vi "1.vi"() -> ()   [LabVIEW 2015]
panel:
  out "数据":string
  in  "文件路径":path
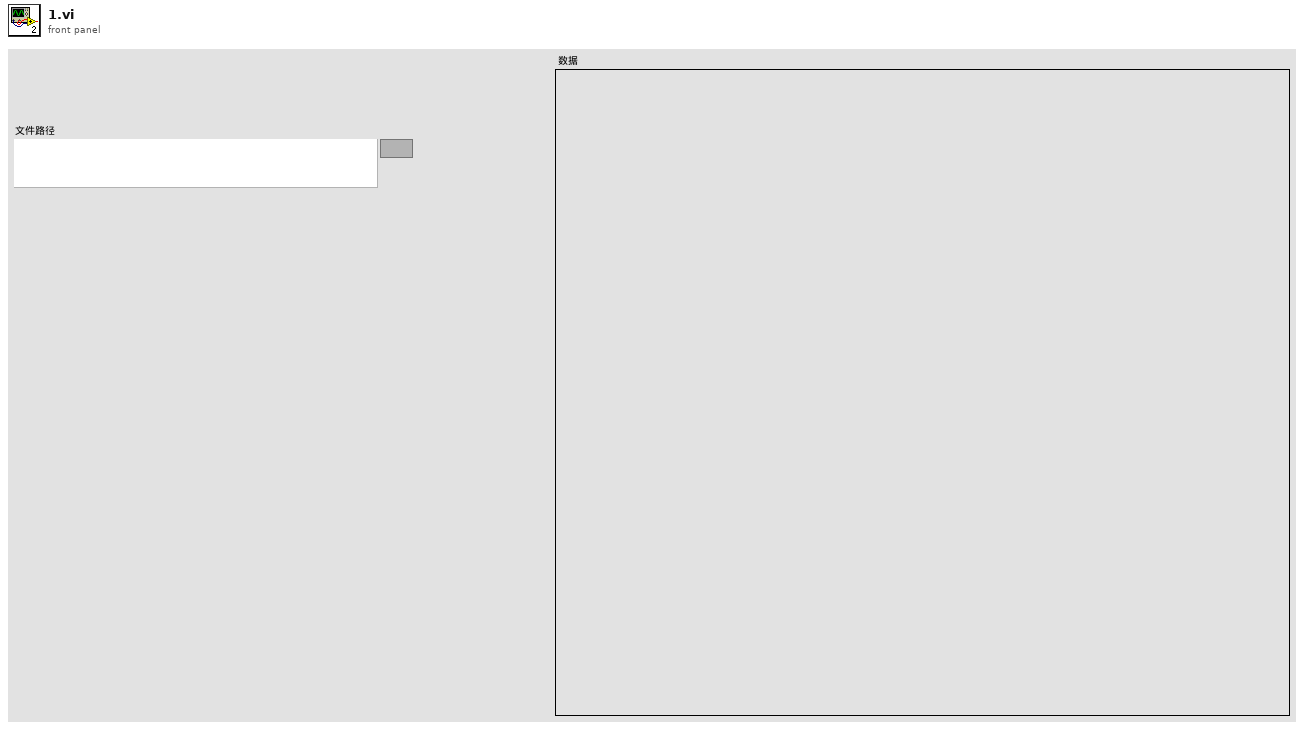
[diagram p1: front panel]
types:
  T1 = enum16{"open", "replace", "create", "open or create", "replace or create", "replace or create with confirmation"}
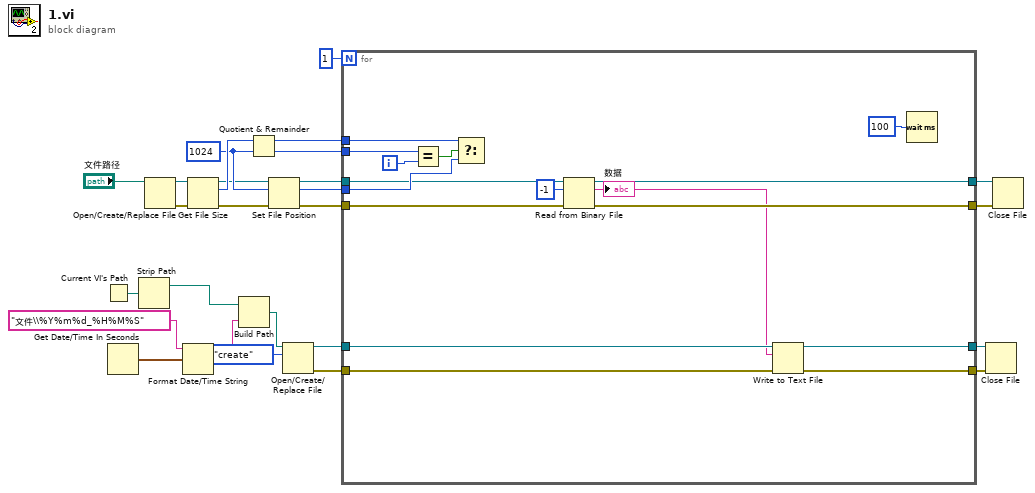
[diagram p0: block diagram]
diagram:
  w19 = 1024 ("y")
  n1 = Current VI's Path() -> (path=w9:path)
  n2 = Get Date/Time In Seconds() -> (seconds since 1Jan1904=w10:timestamp)
  n3 = Strip Path(path=w9) -> (stripped path=w8:path)  [unwired: 1 out]
  n4 = Open/Create/Replace File(file path (use dialog)="文件路径") -> (refnum out=w21:refnum<file>, error out=w22:errorcluster)  [unwired: 5 in, 1 out]
  n5 = Format Date/Time String(time format string (%c)="文件\\%Y%m%d_%H%M%S" ("时间格式字符串(%c)"), seconds (now)=w10) -> (date/time string=w7:string)  [unwired: 1 in]
  n6 = Get File Size(file=w21, error in=w22) -> (refnum out=w14:refnum<file>, size (in bytes)=w20:i64, 0:w13:errorcluster)
  n7 = Build Path(base path=w8, name or relative path=w7) -> (appended path=w6:path)
  n8 = Quotient & Remainder(x=w20, y=w19) -> (x-y*floor(x/y)=w17:i64, floor(x/y)=w18:i64)
  n9 = Set File Position(refnum=w14, error in=w13) -> (refnum out=w12:refnum<file>, error out=w11:errorcluster)  [unwired: 2 in]
  n10 = Open/Create/Replace File(file path (use dialog)=w6, operation (0:open)=T1."create" ("操作(0:open)")) -> (refnum out=w3:refnum<file>, error out=w2:errorcluster)  [unwired: 4 in, 1 out]
  n11 = for {
    N: 1 -> [_]
    tunnel: w12 -> [w28]
    tunnel: w11 -> [w27]
    tunnel: [w41] -> w25
    tunnel: [w40] -> w24
    tunnel: w19 -> [w35]
    tunnel: w18 -> [w39]
    tunnel: w17 -> [w36]
    tunnel: [w32] -> w15
    tunnel: [w33] -> w16
    tunnel: w3 -> [w31]
    tunnel: w2 -> [w30]
    i -> [w38]
    n12 = Equal?(x=w39, y=w38) -> (x = y?=w37:bool)
    n13 = Select(t=w36, s=w37, f=w35) -> ()  [unwired: 1 out]
    n14 = Read from Binary File(8:w27, 10:-1 ("总数(1)"), 11:w28) -> (0:w40:errorcluster, 2:w29:string, 3:w41:refnum<file>)  [unwired: 3 in, 1 out]
    "数据" <- w29
    n15 = Write to Text File(file (use dialog)=w31, text=w29, error in=w30) -> (refnum out=w32:refnum<file>, error out=w33:errorcluster)  [unwired: 1 in, 1 out]
    n16 = Wait (ms)(milliseconds to wait=u32 100 ("等待时间（毫秒）")) -> ()  [unwired: 1 out]
  }
  n17 = Close File(refnum=w15, error in=w16) -> ()  [unwired: 2 out]
  n18 = Close File(refnum=w25, error in=w24) -> ()  [unwired: 2 out]
